vi "UHR-Fleezers Control (host) -Leonardo 04-2018 V2_sym.vi"(0 "Tab Control":T5(tab)=enum."Trap Control (RF)") -> ()   [LabVIEW 2013] (continued)
                    n952 = call "Write to pump.vi"("string"="start", "VISA resource name"=w1530) -> ()  [unwired: 1 out]
                  }
                  frame #3 {
                    n953 = Wait (ms)(milliseconds to wait=u32 500) -> ()  [unwired: 1 out]
                  }
                  frame #4 {
                    n954 = call "Write to pump.vi"("string"="start", "VISA resource name"=w1534) -> ()  [unwired: 1 out]
                  }
                }
              }
            }
          }
          frame Enabled {
            n955 = call "hamilton_controller_shunt2.vi"("Open?"=w1537, "valve"=enum16{"A", "B", "C", "D", "ALL", "E"}."A", "action"=T21."MOVE VALVE") -> ()  [unwired: 8 in, 1 out]
          }
        }
      }
      event "Inject Valve B": Value Change {
        n956 = event-data() -> ()  [unwired: 7 out]
        n957 = disable-structure shown="Enabled" {
          disable-tunnel: "Inject Valve B" -> [w1540 w1560]
          frame Disabled {
            n958 = local read "Pump write delay (ms)"() -> (w1542:dbl)
            n959 = flat-sequence {
              tunnel: w1541 -> [w1555]
              tunnel: w1542 -> [w1551]
              tunnel: w1540 -> [_]
              tunnel: w1542 -> [w1557]
              tunnel: w1541 -> [w1558]
              frame #0 {
                n960 = local read "All Pump Parameters"() -> (w1550:T6)
                n961 = Multiply(x=60.0, y="Flush Center Ch Rate (ul/m)") -> (x*y=w1547:dbl)
                n962 = Unbundle By Name(w1550) -> ("Pump 2"=w1556:T33)
                n963 = call "Set pump parameters.vi"("Pump write delay (ms)"=w1551, "Volume (uL)"="Flush Center Ch Volume (uL)", "Rate (uL/h)"=w1547, "Units"=3.0, "Pump #"=2.0, "Pump Parameters In"=w1556, "VISA resource name"=w1555) -> ("Pump Parameters Out"=w1549:T33)  [unwired: 3 in]
                n964 = Bundle By Name(cluster=w1550, "Pump 2"=w1549) -> (w1548:T6)
                n965 = local write "All Pump Parameters"(w1548) -> ()
                n966 = Add(x="Flush Center Ch Volume (uL)", y="Total Volume\nFlushed (uL)") -> (x+y=w1544:dbl)
                n967 = local write "Total Volume\nFlushed (uL)"(w1544) -> ()
              }
              frame #1 {
                n968 = Wait (ms)(milliseconds to wait=w1557) -> ()  [unwired: 1 out]
              }
              frame #2 {
                n969 = call "Write to pump.vi"("string"="start", "VISA resource name"=w1558) -> ()  [unwired: 1 out]
              }
            }
            n970 = local read "Chemyx Syringe Pump Serial Port"() -> (w1541:refnum<visa-resource-name>)
          }
          frame Enabled {
            n971 = call "hamilton_controller.vi"("Open?"=w1560, "valve"=enum16{"A", "B", "C", "D", "ALL"}."B", "action"=T21."MOVE VALVE") -> ()  [unwired: 8 in, 1 out]
          }
        }
      }
      event "Inject Bottom": Value Change {
        n972 = event-data() -> ()  [unwired: 7 out]
        n973 = call "hamilton_controller_shunt2.vi"("Open?"="Inject Bottom", "valve"=enum16{"A", "B", "C", "D", "ALL", "E"}."C", "action"=T21."MOVE VALVE") -> ()  [unwired: 8 in, 1 out]
      }
      event "Shunt:": Value Change {
        n974 = event-data() -> ()  [unwired: 7 out]
        n975 = call "hamilton_controller_shunt2.vi"("Open?"="Shunt:", "valve"=enum16{"A", "B", "C", "D", "ALL", "E"}."D", "action"=T21."MOVE VALVE") -> ()  [unwired: 8 in, 1 out]
      }
      event "Shunt 2:   2": Value Change {
        n976 = event-data() -> ()  [unwired: 7 out]
        n977 = call "hamilton_controller_shunt2.vi"("Open?"="Shunt 2:   2", "valve"=enum16{"A", "B", "C", "D", "ALL", "E"}."E", "action"=T21."MOVE VALVE") -> ()  [unwired: 8 in, 1 out]
      }
      event "Flip Green Filter": Value Change {
        n978 = event-data() -> ()  [unwired: 7 out]
        n979 = local write "Flip Green Filter"("Flip Green Filter") -> ()
        n980 = flat-sequence {
          tunnel: w1579 -> [w1584]
          tunnel: w1578 -> [w1583]
          tunnel: [w1581] -> w1576
          tunnel: [w1580] -> w1575
          tunnel: [w1586] -> w1574
          tunnel: w1576 -> [w1586]
          tunnel: [w1585] -> w1573
          tunnel: w1575 -> [w1585]
          tunnel: w1574 -> [w1590]
          tunnel: w1573 -> [w1589]
          tunnel: [w1588] -> w1577
          frame #0 {
            n981 = xnode "Read/Write Control"("FPGA VI Reference In"=w1584, "error in"=w1583, "Green Filter Flipper"=TRUE) -> ("FPGA VI Reference Out"=w1581:T20, "error out"=w1580:errorcluster)
          }
          frame #1 {
            n982 = Wait (ms)(milliseconds to wait=u32 100) -> ()  [unwired: 1 out]
          }
          frame #2 {
            n983 = xnode "Read/Write Control"("FPGA VI Reference In"=w1590, "error in"=w1589, "Green Filter Flipper"=FALSE) -> ("error out"=w1588:errorcluster)  [unwired: 1 out]
          }
        }
      }
      event "Pump 1 contents", "Pump 3 contents": Value Change {
        n984 = event-data() -> ()  [unwired: 7 out]
        n985 = local read "Pump 1 contents"() -> (→"Pump 1 cont disp":string)
        n986 = local read "Pump 3 contents"() -> (→"Pump 3 cont disp":string)
      }
      event "Reset Trap Pos. FB": Value Change {
        n987 = event-data() -> ()  [unwired: 7 out]
        n988 = xnode "Read/Write Control"("FPGA VI Reference In"=w1596, "error in"=w1595, "Trap Pos. FB Reset"="Reset Trap Pos. FB") -> ()  [unwired: 2 out]
      }
      event "Trap Pos. FB ON": Value Change {
        n989 = event-data() -> ()  [unwired: 7 out]
        n990 = xnode "Read/Write Control"("FPGA VI Reference In"=w1611, "error in"=w1610) -> ("FPGA VI Reference Out"=w1608:T20, "BD1 Frequency Out 1"=w1605:u64)  [unwired: 1 out]
        n991 = To Double Precision Float(number=w1605) -> (double precision float=w1604:dbl)
        n992 = Multiply(x=49125000.0, y=6.0) -> (x*y=w1603:dbl)
        n993 = Multiply(x=w1604, y=w1603) -> (x*y=w1601:dbl)
        n994 = Scale By Power Of 2(n=-48, x=w1601) -> (x*2^n=w1600:dbl)
        n995 = Divide(x=w1600, y=1000000.0) -> (x/y=w1597:dbl)
        n996 = flat-sequence {
          tunnel: [w1614] -> w1609
          tunnel: w1608 -> [w1615]
          tunnel: w1605 -> [w1613]
          tunnel: "Trap Pos. FB ON" -> [w1612]
          tunnel: "Trap Pos. FB ON" -> [w1621]
          tunnel: w1609 -> [w1620]
          tunnel: "Trap Pos. FB ON" -> [w1623]
          tunnel: w1597 -> [w1622]
          frame #0 {
            n997 = case shown="False" w1612 {
              tunnel: w1615 -> [w1618 w1619]
              tunnel: [w1617 w1619] -> w1614
              tunnel: w1613 -> [w1616 _]
              frame False {
                n998 = xnode "Read/Write Control"("FPGA VI Reference In"=w1618, "BD 1 Frequency 1"=w1616) -> ("FPGA VI Reference Out"=w1617:T20)  [unwired: 1 in, 1 out]
              }
              frame True {
              }
            }
          }
          frame #1 {
            n999 = xnode "Read/Write Control"("FPGA VI Reference In"=w1620, "Force feedback"=w1621) -> ()  [unwired: 1 in, 2 out]
          }
          frame #2 {
            n1000 = case shown="False" w1623 {
              tunnel: w1622 -> [w1626 _]
              frame False {
                n1001 = local read "T2 for asymmetric\n(MHz)"() -> (w1624:dbl)
                n1002 = Subtract(x=w1624, y=w1626) -> (x-y=w1625:dbl)
                n1003 = property on="Trap Delta (MHz)" class="DigNum (strict)"("Val(Sgnl)"=w1625) -> ()  [unwired: 2 in, 2 out]
              }
              frame True {
              }
            }
          }
        }
      }
      event "Diff. FB.", "Trap Pos. FB Gains", "Trap Pos. FB Mult Factor", "Trap Pos. FB Offset Factor", "Trap Pos FB Negate Action", "Trap Pos FB Monitor\nT1 or T2", "Negate Diff?": Value Change {
        n1004 = event-data() -> ()  [unwired: 7 out]
        n1005 = xnode "Read/Write Control"("FPGA VI Reference In"=w1637, "error in"=w1636, "Trap pos. FB Range"="Trap Pos. FB Range", "Trap Pos. FB Gains"="Trap Pos. FB Gains", "Trap Pos. FB Mult Factor"="Trap Pos. FB Mult Factor", "Trap Pos. FB Offset Factor"="Trap Pos. FB Offset Factor", "Trap Pos FB Negate Action"="Trap Pos FB Negate Action", "Trap Pos FB Monitor T1 or T2"="Trap Pos FB Monitor\nT1 or T2", "AI1 X Scale"="Trap Pos. AI1 X Pre-scale", "Negate Diff?"="Negate Diff?", "Diff FB Measurement?"="Diff. FB.") -> ()  [unwired: 2 out]
      }
      event "Trap Pos FB SP": Value Change {
        n1006 = event-data() -> ()  [unwired: 7 out]
        n1007 = xnode "Read/Write Control"("FPGA VI Reference In"=w1640, "error in"=w1639, "Trap Pos. FB SP"="Trap Pos FB SP") -> ()  [unwired: 2 out]
        n1008 = disable-structure shown="Disabled" {
          frame Disabled {
            n1009 = local read "Trap X AI1 (DMA)"() -> (w1661:T13)
            n1010 = local read "Trap X (AI1)"() -> (w1662:T1)
            n1011 = local read "Setpoint offset\nCorrection values"() -> (w1655:dbl[])
            n1012 = local read "Trap Delta (MHz)"() -> (w1659:dbl)
            n1013 = local read "B factor"() -> (w1646:dbl)
            n1014 = Unbundle(w1662) -> ("Trap 1"=w1660:fxp<+/-,16,1>, "Trap 2"=w1649:fxp<+/-,16,1>)
            n1015 = Unbundle(w1661) -> ("Set 1"=w1645:fxp<+/-,16,1>, "Set 2"=w1644:fxp<+/-,16,1>)
            n1016 = Negate(x=w1649) -> (-x=w1642:fxp<+/-,17,2>)
            n1017 = Negate(x=w1660) -> (-x=w1643:fxp<+/-,17,2>)
            n1018 = Divide(x=w1659, y=0.1) -> (x/y=w1657:dbl)
            n1019 = Multiply(x=w1644, y=w1646) -> (x*y=w1647:dbl)
            n1020 = Subtract(x=w1645, y=w1647) -> (x-y=w1652:dbl)
            n1021 = To Long Integer(number=w1657) -> (32bit integer=w1656:i32)
            n1022 = Index Array(array=w1655, index=w1656) -> (element=w1651:dbl)
            n1023 = Multiply(x=w1646, y=w1642) -> (x*y=w1648:dbl)
            n1024 = Subtract(x=w1643, y=w1648) -> (x-y=w1654:dbl)
            n1025 = Add(x=w1654, y=w1651) -> (x+y=→"ideal setpoint fpga":dbl)
            n1026 = Add(x=w1652, y=w1651) -> (x+y=→"ideal setpoint avgd":dbl)
          }
          frame Enabled {
          }
        }
        n1027 = disable-structure shown="Enabled" {
          frame Enabled {
          }
          frame Disabled {
            n1028 = local write "B factor"(1.0 ("B factor")) -> ()
          }
        }
      }
      event "Simulate stepping": Value Change {
        n1029 = event-data() -> ()  [unwired: 7 out]
        n1030 = flat-sequence {
          tunnel: w1664 -> [w1667]
          tunnel: [w1666] -> _
          tunnel: w1663 -> [w1665]
          frame #0 {
            n1031 = while {
              tunnel: w1667 -> [w1695]
              tunnel: [w1694] -> w1666 mode=indexing
              tunnel: w1665 -> [w1693]
              i -> [w1679]
              stop <- w1676 stop-if-true
              w1669 = 1000.0
              n1032 = Divide(x="Backtrack probability", y=100) -> (x/y=w1703:dbl)
              n1033 = Random Number (0-1)() -> (number: 0 to 1=w1704:dbl)
              n1034 = Greater?(x=w1704, y=w1703) -> (0:w1702:bool)
              n1035 = Select(t=1, s=w1702, f=-1) -> (s? t:f=w1699:i32)
              n1036 = local read "BD 1 Frequency 2 (MHz)"() -> (w1674:dbl)
              n1037 = Multiply(x=w1699, y="Step size (nm)") -> (x*y=w1697:dbl)
              "Step taken" <- w1697
              n1038 = Divide(x=w1697, y=168.33) -> (x/y=w1672:dbl)
              n1039 = local read "BD 1 Frequency 1 (MHz)"() -> (w1673:dbl)
              n1040 = local read "X RF Frequency Limits (MHz)"() -> (w1692:T16)
              n1041 = local read "Y RF Frequency Limits (MHz)"() -> (w1691:T16)
              n1042 = Subtract(x=w1673, y=w1672) -> (x-y=w1671:dbl)
              n1043 = local write "BD 1 Frequency 1 (MHz)"(w1671) -> ()
              n1044 = local read "BD 2 Frequency 1 (MHz)"() -> (w1689:dbl)
              n1045 = local read "BD 2 Frequency 2 (MHz)"() -> (w1690:dbl)
              n1046 = call "set RF board frequency - interlace.vi"("Board 2 Frequency Limits"=w1691, "Board 1 Frequency Limits"=w1692, "error in"=w1695, "FPGA VI Reference In"=w1693, "Board 2 Frequency 2 (MHz)"=w1690, "Board 2 Frequency 1 (MHz)"=w1689, "Board 1 Frequency 2 (MHz)"=w1674, "Board 1 Frequency 1  (MHz)"=w1671) -> ("error out"=w1694:errorcluster)  [unwired: 2 in, 1 out]
              n1047 = Subtract(x=w1674, y=w1671) -> (x-y=w1688:dbl)
              n1048 = Subtract(x=w1690, y=w1689) -> (x-y=w1687:dbl)
              n1049 = Square(x=w1687) -> (x^2=w1685:dbl)
              n1050 = Square(x=w1688) -> (x^2=w1686:dbl)
              n1051 = Add(x=w1686, y=w1685) -> (x+y=w1684:dbl)
              n1052 = Square Root(x=w1684) -> (sqrt(x)=w1675:dbl)
              n1053 = local write "Trap Delta (MHz)"(w1675) -> ()
              n1054 = property on="Initial delta (MHz)" class="DigNum (strict)"("Val(Sgnl)"=w1675) -> ()  [unwired: 2 in, 2 out]
              n1055 = Multiply(x="Mean dwell time (s)", y=w1669) -> (x*y=w1681:dbl)
              n1056 = case shown="\"Gamma2\"" "Distribution" {
                tunnel: w1681 -> [w1708 w1712 w1715]
                tunnel: [w1708 w1709 w1716] -> w1670
                frame "uniform", Default {
                }
                frame "Exponential" {
                  n1057 = call-poly <vilib>:"Continuous Random.vi"("b"=w1712, "samples"=1) -> ("exp random data"=w1710:dbl[])  [unwired: 8 in, 1 out]
                  n1058 = Index Array(array=w1710) -> (element=w1709:dbl)  [unwired: 1 in]
                }
                frame "Gamma2" {
                  w1713 = 2.0
                  # "Note: the shape and scale\nparameters of the gamma\nare inverted because LabView..."
                  n1059 = Divide(x=w1715, y=w1713) -> (x/y=w1714:dbl)
                  n1060 = call-poly <vilib>:"Continuous Random.vi"("c"=w1714, "b"=w1713, "samples"=1) -> ("gamma random numbers"=w1717:dbl[])  [unwired: 7 in, 1 out]
                  n1061 = Index Array(array=w1717) -> (element=w1716:dbl)  [unwired: 1 in]
                }
              }
              n1062 = Divide(x=w1670, y=w1669) -> (x/y=→"Step duration":dbl)
              n1063 = To Unsigned Long Integer(number=w1670) -> (unsigned 32bit integer=w1682:u32)
              n1064 = Add(x=w1679, y=1) -> (x+y=w1678:i32)
              n1065 = Wait (ms)(milliseconds to wait=w1682) -> ()  [unwired: 1 out]
              n1066 = Equal?(x=w1678, y="Number of steps") -> (x = y?=w1676:bool)
            }
          }
          frame #1 {
            n1067 = local write "Simulate stepping"(FALSE) -> ()
          }
        }
      }
      event "Set SP to Reading": Value Change {
        n1068 = event-data() -> ()  [unwired: 7 out]
        n1069 = local read "Trap Pos FB Monitor\nT1 or T2"() -> (w1727:bool)
        n1070 = local read "Trap X AI1 (DMA)"() -> (w1730:T13)
        n1071 = local read "Trap X (AI1)"() -> (w1733:T1)
        n1072 = Unbundle By Name(w1733) -> ("Trap 1"=w1732:fxp<+/-,16,1>, "Trap 2"=w1731:fxp<+/-,16,1>)
        n1073 = Unbundle By Name(w1730) -> ("Set 1"=w1729:fxp<+/-,16,1>, "Set 2"=w1728:fxp<+/-,16,1>)
        n1074 = Select(t=w1732, s=w1727, f=w1731) -> (s? t:f=w1726:fxp<+/-,16,1>)
        n1075 = Select(t=w1729, s=w1727, f=w1728) -> (s? t:f=w1725:fxp<+/-,16,1>)
        n1076 = Not(x="Set SP Using...") -> (.not. x?=w1720:bool)
        n1077 = Select(t=w1726, s=w1720, f=w1725) -> (s? t:f=w1721:fxp<+/-,16,1>)
        n1078 = xnode "Read/Write Control"("FPGA VI Reference In"=w1723, "error in"=w1722, "Trap Pos. FB SP"=w1721) -> ()  [unwired: 2 out]
        n1079 = local write "Trap Pos FB SP"(w1721) -> ()
      }
      event "Trap Pos. FB Out Scale 2^n": Value Change {
        n1080 = event-data() -> ()  [unwired: 7 out]
        n1081 = Scale By Power Of 2(n="Trap Pos. FB Out Scale 2^n", x=ext 1.0) -> (x*2^n=w1735:ext)
        n1082 = property on="Trap Pos. FB Mult Factor" class="DigNum (strict)"("Val(Sgnl)"=w1735) -> ()  [unwired: 2 in, 2 out]
      }
      event "Trap Pos FB Int Count": Value Change {
        n1083 = event-data() -> ()  [unwired: 7 out]
        n1084 = xnode "Read/Write Control"("FPGA VI Reference In"=w1740, "error in"=w1739, "Trap Pos FB Int Count"="Trap Pos FB Int Count") -> ()  [unwired: 2 out]
      }
      event "Target Force (pN)", "Setpoint offset\nCorrection values", "Raster target force (pN)": Value Change {
        w1749 = 2.0
        n1085 = event-data() -> ()  [unwired: 7 out]
        n1086 = disable-structure "Removed B Factor to improve position feedback - Alex 081418 1of3" shown="Enabled" {
          disable-tunnel: [w1779 fxp<+/-,32,16> 1.0 ("B factor")] -> w1741
          frame Disabled {
            n1087 = local read "B factor"() -> (w1780:dbl)
            n1088 = To Fixed-Point(number=w1780) -> (fixed-point=w1779:fxp<+/-,16,16>)  [unwired: 1 in]
          }
          frame Enabled {
          }
        }
        n1089 = xnode "Read/Write Control"("FPGA VI Reference In"=w1743, "B factor"=w1741) -> ("BD1 Frequency Out 1"=w1770:u64)  [unwired: 1 in, 2 out]
        n1090 = local read "BD 1 Frequency 2 (MHz)"() -> (w1769:dbl)
        n1091 = local read "Target Force (pN)"() -> (w1755:dbl)
        n1092 = To Double Precision Float(number=w1770) -> (double precision float=w1776:dbl)
        n1093 = Multiply(x=49125000.0, y=6.0) -> (x*y=w1775:dbl)
        n1094 = Multiply(x=w1776, y=w1775) -> (x*y=w1773:dbl)
        n1095 = Scale By Power Of 2(n=-48, x=w1773) -> (x*2^n=w1772:dbl)
        n1096 = Divide(x=w1772, y=1000000.0) -> (x/y=w1768:dbl)
        n1097 = Subtract(x=w1769, y=w1768) -> (x-y=w1767:dbl)
        n1098 = local read "T1 kappa_x (pN/nm)"() -> (w1756:dbl)
        n1099 = local read "T1 alpha_x (nm/V)"() -> (w1757:dbl)
        n1100 = local read "Negate offset difference"() -> (w1758:bool)
        n1101 = local read "Offset file step size"() -> (w1766:dbl)
        n1102 = Multiply(x="Raster target force (pN)", y=w1749) -> (x*y=w1748:dbl)
        n1103 = Multiply(x=w1755, y=w1749) -> (x*y=w1754:dbl)
        n1104 = local read "Setpoint offset\nCorrection values"() -> (w1763:dbl[])
        n1105 = Divide(x=w1767, y=w1766) -> (x/y=w1765:dbl)
        n1106 = Select(t=-1, s=w1758, f=1) -> (s? t:f=w1759:i32)
        n1107 = To Long Integer(number=w1765) -> (32bit integer=w1764:i32)
        n1108 = Multiply(x=w1757, y=w1756) -> (x*y=w1747:dbl)
        n1109 = Divide(x=w1754, y=w1747) -> (x/y=w1753:dbl)
        n1110 = Index Array(array=w1763, index=w1764) -> (element=w1762:dbl)
        n1111 = Divide(x=w1748, y=w1747) -> (x/y=w1746:dbl)
        n1112 = Multiply(x=w1759, y=w1762) -> (x*y=w1745:dbl)
        n1113 = Add(x=w1753, y=w1745) -> (x+y=w1752:dbl)
        n1114 = Add(x=w1746, y=w1745) -> (x+y=w1744:dbl)
        n1115 = To Fixed-Point(number=w1744) -> (fixed-point=w1742:fxp<+/-,16,1>)  [unwired: 1 in]
        n1116 = To Fixed-Point(number=w1752) -> (fixed-point=w1751:fxp<+/-,16,1>)  [unwired: 1 in]
        n1117 = property on="Trap Pos FB SP" class="DigNum (strict)"("Val(Sgnl)"=w1751) -> ()  [unwired: 2 in, 2 out]
        n1118 = xnode "Read/Write Control"("FPGA VI Reference In"=w1743, "Raster setpoint"=w1742) -> ()  [unwired: 1 in, 2 out]
      }
      event "Read setpoint correction\nfile": Value Change {
        n1119 = event-data() -> ()  [unwired: 7 out]
        n1120 = local write "Read setpoint correction\nfile"(FALSE) -> ()
        n1121 = Open/Create/Replace File(file path (use dialog)="Setpoint correction\noffset file", operation (0:open)=T24."open", access (0:read/write)=enum16{"read/write", "read-only", "write-only"}."read-only") -> (refnum out=w1807:refnum<file>)  [unwired: 1 in, 4 out]
        n1122 = Deny Access(7:w1807) -> (3:w1805:refnum<file>)  [unwired: 1 in, 2 out]
        n1123 = Read from Binary File(5:0.0, 9:T30."big-endian, network order" ("byte order (0:big-endian, network order)"), 10:-1 ("count (1)"), 11:w1805) -> (2:w1798:dbl[], 3:w1804:refnum<file>)  [unwired: 1 in, 3 out]
        n1124 = Close File(refnum=w1804) -> ()  [unwired: 1 in, 2 out]
        n1125 = Index Array(array=w1798, index=0) -> (element=w1794:dbl)
        n1126 = local write "Offset file step size"(w1794) -> ()
        n1127 = Array Subset(array=w1798, index=3) -> (w1797:dbl[])  [unwired: 1 in]
        n1128 = local read "T1 kappa_x (pN/nm)"() -> (w1792:dbl)
        n1129 = local read "T1 alpha_x (nm/V)"() -> (w1793:dbl)
        n1130 = local read "T2 alpha_x (nm/V)"() -> (w1791:dbl)
        n1131 = local read "T2 kappa_x (pN/nm)"() -> (w1790:dbl)
        n1132 = Decimate 1D Array(w1797) -> (w1786:dbl[], w1787:dbl[])  [unwired: 1 out]
        n1133 = local read "Offset Values"() -> (w1796:T14)
        n1134 = Multiply(x=w1793, y=w1792) -> (x*y=w1788:dbl)
        n1135 = Multiply(x=w1791, y=w1790) -> (x*y=w1789:dbl)
        n1136 = Bundle By Name(cluster=w1796, "Trap 1X offset"=w1786, "Trap 2X offset"=w1787) -> (w1795:T14)
        n1137 = Divide(x=w1789, y=w1788) -> (x/y=w1783:dbl)
        n1138 = disable-structure "Removed B Factor to better position FB - Alex 081418 3of3" shown="Enabled" {
          disable-tunnel: w1783 -> [w1811 _]
          disable-tunnel: [w1811 1.0] -> w1782
          frame Disabled {
          }
          frame Enabled {
          }
        }
        n1139 = Multiply(x=w1787, y=w1782) -> (x*y=w1785:dbl[])
        n1140 = local write "Offset Values"(w1795) -> ()
        n1141 = Subtract(x=w1786, y=w1785) -> (x-y=w1784:dbl[])
        n1142 = property on="B factor" class="DigNum (strict)"("Val(Sgnl)"=w1782) -> ()  [unwired: 2 in, 2 out]
        n1143 = property on="Setpoint offset\nCorrection values" class="Arr (strict)"("Val(Sgnl)"=w1784) -> ()  [unwired: 2 in, 2 out]
      }
      event "MCL Tracking": Value Change {
        n1144 = event-data() -> ()  [unwired: 7 out]
        n1145 = case shown="True" "MCL Tracking" {
          frame False {
            n1146 = local read "Current MCL (V)"() -> (w1814:dbl)
            n1147 = local write "AO2"(w1814) -> ()
          }
          frame True {
            n1148 = local read "BD 1 Frequency 1 (MHz)"() -> (→"Zero T1 position":dbl)
            n1149 = local read "AO2"() -> (→"Zero MCL x position":dbl)
          }
        }
      }
      event "Scale intensities": Value Change {
        n1150 = event-data() -> ()  [unwired: 7 out]
        n1151 = local read "Trap Intensity\nSetpoints (V)"() -> (w1820:cluster{"Set 1":dbl, "Set 2":dbl})
        n1152 = local read "T1 kappa_x (pN/nm)"() -> (w1826:dbl)
        n1153 = local read "T2 kappa_x (pN/nm)"() -> (w1825:dbl)
        n1154 = Unbundle By Name(w1820) -> ("Set 1"=w1822:dbl, "Set 2"=w1821:dbl)
        n1155 = case shown="True" "Scale intensities" {
          tunnel: "Scale factor" -> [w1836 w1848]
          tunnel: "Scale factor" -> [w1831 w1841]
          tunnel: w1826 -> [w1838 w1847]
          tunnel: w1825 -> [w1837 w1846]
          tunnel: [w1834 w1845] -> w1824
          tunnel: [w1835 w1844] -> w1823
          tunnel: w1822 -> [w1833 w1843]
          tunnel: w1821 -> [w1832 w1842]
          tunnel: [w1830 w1840] -> w1819
          tunnel: [w1829 w1839] -> w1818
          frame False {
            n1156 = Divide(x=w1838, y=w1831) -> (x/y=w1834:dbl)
            n1157 = Divide(x=w1837, y=w1836) -> (x/y=w1835:dbl)
            n1158 = Divide(x=w1833, y=w1831) -> (x/y=w1830:dbl)
            n1159 = Divide(x=w1832, y=w1831) -> (x/y=w1829:dbl)
          }
          frame True {
            n1160 = Multiply(x=w1843, y=w1841) -> (x*y=w1840:dbl)
            n1161 = Multiply(x=w1842, y=w1841) -> (x*y=w1839:dbl)
            n1162 = Multiply(x=w1847, y=w1841) -> (x*y=w1845:dbl)
            n1163 = Multiply(x=w1848, y=w1846) -> (x*y=w1844:dbl)
          }
        }
        n1164 = local write "T2 kappa_x (pN/nm)"(w1823) -> ()
        n1165 = local write "T1 kappa_x (pN/nm)"(w1824) -> ()
        n1166 = Bundle By Name(cluster=w1820, "Set 1"=w1819, "Set 2"=w1818) -> (w1817:cluster{"Set 1":dbl, "Set 2":dbl})
        n1167 = property on="Trap Intensity\nSetpoints (V)" class="Clust (strict)"("Val(Sgnl)"=w1817) -> ()  [unwired: 2 in, 2 out]
      }
    }
    "error out 2" <- w772
    n1168 = node-c288() -> ()  [unwired: 1 in, 1 out]
  }
  n1169 = node-c288() -> (w103:T25)  [unwired: 4 in]
  n1170 = timed-loop "Run Scripts, including: stage motion" {
    timing: w103 -> [_]
    timing-out: [_] -> w102
    tunnel: w61 -> [_]
    stop <- w1850 stop-if-true
    n1171 = node-c288() -> ()  [unwired: 1 in, 1 out]
    n1172 = event shown="[8] \"Take Stepping Data\": Value Change" {
      selector: _ -> [_ _ _ _ _ _ _ _ _ _ _ _]
      dyn-events: _ -> [_ _ _ _ _ _ _ _ _ _ _ _]
      timeout: 50 -> [_ _ _ _ _ _ _ _ _ _ _ _]
      tunnel: ["Move Cap. 1 (DNA Top)" _ "Cal/Data Acq. Spot" "Dump Beads" "Dip for Protein" _ "Got ADig bead" "Got DNA bead" "Take Stepping Data" _ "Take Detection Laser\nImage" _] -> _
      tunnel: [_ _ _ _ _ _ _ _ _ _ _ w2060] -> w1850
      event "Move Cap. 1 (DNA Top)": Value Change {
        n1173 = event-data() -> ()  [unwired: 1 in, 5 out]
        n1174 = local write "Move Cap. 1 (DNA Top)"(FALSE ("Move Cap. 1 (DNA Right)")) -> ()
        n1175 = flat-sequence {
          tunnel: "Cap 1 Samp Flow ON" -> [w1856]
          frame #0 {
            n1176 = local write "Stage Moving"(FALSE ("Stage Moving")) -> ()
            n1177 = case "stop flow" shown="True" w1856 {
              frame False {
              }
              frame True {
                n1178 = call "hamilton_controller.vi"("Open?"=FALSE, "valve"=enum16{"A", "B", "C", "D", "ALL"}."C", "action"=T21."MOVE VALVE") -> ()  [unwired: 8 in, 1 out]
              }
            }
            n1179 = case shown="True" TRUE {
              tunnel: "Cap 1 T ON" -> [w1865 w1866]
              frame False {
                n1180 = property on="Trap 1 (ON/OFF)" class="Bool (strict)"("Val(Sgnl)"=w1865) -> ()  [unwired: 2 in, 2 out]
              }
              frame True {
                n1181 = property on="Trap 2 (ON/OFF)" class="Bool (strict)"("Val(Sgnl)"=w1866) -> ()  [unwired: 2 in, 2 out]
              }
            }
            n1182 = call <vilib>:"Beep.vi"() -> ()  [unwired: 3 in, 9 out]
            n1183 = case shown="True" "Cap 1 Flow ON" {
              frame False {
              }
              frame True {
                n1184 = property on="Main:" class="Bool (strict)"("Val(Sgnl)"=TRUE ("Value (Signaling)")) -> ()  [unwired: 2 in, 2 out]
              }
            }
          }
        }
      }
      event Timeout {
        n1185 = event-data() -> ()  [unwired: 1 in, 2 out]
      }
      event "Cal/Data Acq. Spot": Value Change {
        # "wait for calibration file\nto be written"
        # "signal save cal true\nthis tells the data \nacquisition loop to\nstart sending the data\nto a calibration file"
        # "separate traps to\nthe desired trap delta"
        # "move stage to data acquisition spot"
        # "CHANGE FISH FOR TETHER BACK\nTO TRUE VALUE HERE."
        n1186 = event-data() -> ()  [unwired: 1 in, 5 out]
        n1187 = flat-sequence {
          tunnel: ["Cal @ (MHz)"] -> w1867
          tunnel: w1867 -> [w1879]
          tunnel: w1867 -> [w1900]
          frame #0 {
            n1188 = property on="Trap Delta (MHz)" class="DigNum (strict)"("Val(Sgnl)"="Cal @ (MHz)") -> ()  [unwired: 2 in, 2 out]
            n1189 = call <vilib>:"Beep.vi"() -> ()  [unwired: 3 in, 9 out]
          }
          frame #1 {
            n1190 = local read "Scale intensities"() -> (w1871:bool)
            n1191 = case shown="True" w1871 {
              frame False {
              }
              frame True {
                n1192 = property on="Scale intensities" class="Bool (strict)"("Val(Sgnl)"=FALSE ("Value (Signaling)")) -> ()  [unwired: 2 in, 2 out]
              }
            }
          }
          frame #2 {
            n1193 = Wait (ms)(milliseconds to wait=u32 500) -> ()  [unwired: 1 out]
          }
          frame #3 {
            n1194 = property on="Save Calibration" class="Bool (strict)"("Val(Sgnl)"=TRUE ("Value (Signaling)")) -> ()  [unwired: 2 in, 2 out]
          }
          frame #4 {
            n1195 = Wait (ms)(milliseconds to wait=u32 4000) -> ()  [unwired: 1 out]
          }
          frame #5 {
            n1196 = while {
              stop <- w1876 stop-if-true
              n1197 = local read "Saving..."() -> (w1877:bool)
              n1198 = Wait (ms)(milliseconds to wait=u32 100) -> ()  [unwired: 1 out]
              n1199 = Not(x=w1877) -> (.not. x?=w1876:bool)
            }
          }
          frame #6 {
            n1200 = case shown="True" "W/ Offset 1" {
              tunnel: w1879 -> [_ w1881]
              frame False {
              }
              frame True {
                n1201 = stacked-sequence {
                  tunnel: w1881 -> [_ _ _ _ _ _ _ w1898]
                  frame #0 {
                    n1202 = Replace Array Subset(array=u32[] [0] ("Index Values"), new element="Offset 1 Set", index=0) -> (w1882:u32[])
                    n1203 = property on="Saved AOD Raster Scan Parameter Sets" class="Arr (strict)"("Index Values"=w1882) -> ()  [unwired: 2 in, 2 out]
                    n1204 = property on="Trap Delta (MHz)" class="DigNum (strict)"("Val(Sgnl)"="Offset 1 Start (MHz)") -> ()  [unwired: 2 in, 2 out]
                  }
                  frame #1 {
                    n1205 = Wait (ms)(milliseconds to wait=u32 200) -> ()  [unwired: 1 out]
                  }
                  frame #2 {
                    n1206 = property on="Load parameters" class="Bool (strict)"("Val(Sgnl)"=TRUE ("Value (Signaling)")) -> ()  [unwired: 2 in, 2 out]
                  }
                  frame #3 {
                    n1207 = Wait (ms)(milliseconds to wait=u32 200) -> ()  [unwired: 1 out]
                  }
                  frame #4 {
                    n1208 = property on="Trap Raster Scan" class="Bool (strict)"("Val(Sgnl)"=TRUE ("Value (Signaling)")) -> ()  [unwired: 2 in, 2 out]
                  }
                  frame #5 {
                    n1209 = Wait (ms)(milliseconds to wait=u32 2000) -> ()  [unwired: 1 out]
                  }
                  frame #6 {
                    n1210 = while {
                      stop <- w1895 stop-if-true
                      n1211 = local read "Raster Scanning..."() -> (w1897:bool)
                      n1212 = local read "Saving..."() -> (w1893:bool)
                      n1213 = Wait (ms)(milliseconds to wait=u32 100) -> ()  [unwired: 1 out]
                      n1214 = Not(x=w1893) -> (.not. x?=w1892:bool)
                      n1215 = Not(x=w1897) -> (.not. x?=w1894:bool)
                      n1216 = And(x=w1894, y=w1892) -> (x .and. y?=w1895:bool)
                    }
                  }
                  frame #7 {
                    n1217 = property on="Trap Delta (MHz)" class="DigNum (strict)"("Val(Sgnl)"=w1898) -> ()  [unwired: 2 in, 2 out]
                  }
                }
              }
            }
          }
          frame #7 {
            n1218 = local read "Save ave N"() -> (w1899:dbl)
            n1219 = case shown="True" "W/ Offset 2" {
              tunnel: w1900 -> [_ w1906]
              tunnel: w1899 -> [_ w1905]
              frame False {
                n1220 = Multiply(x="Cal read wait (s)", y=u32 1000 ("milliseconds to wait")) -> (x*y=w1903:u32)
                n1221 = Wait (ms)(milliseconds to wait=w1903) -> ()  [unwired: 1 out]
              }
              frame True {
                n1222 = stacked-sequence {
                  tunnel: w1906 -> [_ _ _ _ _ _ _ _ _ w1927 _ _]
                  tunnel: w1905 -> [_ _ _ _ _ _ _ _ _ w1925 _ _]
                  frame #0 {
                    n1223 = property on="Save ave N" class="DigNum (strict)"("Val(Sgnl)"=1.0 ("Value (Signaling)")) -> ()  [unwired: 2 in, 2 out]
                  }
                  frame #1 {
                    n1224 = Wait (ms)(milliseconds to wait=u32 500) -> ()  [unwired: 1 out]
                  }
                  frame #2 {
                    n1225 = property on="Trap Delta (MHz)" class="DigNum (strict)"("Val(Sgnl)"="Offset 2 Start (MHz)") -> ()  [unwired: 2 in, 2 out]
                    n1226 = Replace Array Subset(array=u32[] [0] ("Index Values"), new element="Offset 2 Set", index=0) -> (w1911:u32[])
                    n1227 = property on="Saved AOD Raster Scan Parameter Sets" class="Arr (strict)"("Index Values"=w1911) -> ()  [unwired: 2 in, 2 out]
                  }
                  frame #3 {
                    n1228 = Wait (ms)(milliseconds to wait=u32 500) -> ()  [unwired: 1 out]
                  }
                  frame #4 {
                    n1229 = property on="Load parameters" class="Bool (strict)"("Val(Sgnl)"=TRUE ("Value (Signaling)")) -> ()  [unwired: 2 in, 2 out]
                  }
                  frame #5 {
                    n1230 = Wait (ms)(milliseconds to wait=u32 500) -> ()  [unwired: 1 out]
                  }
                  frame #6 {
                    n1231 = property on="Trap Raster Scan" class="Bool (strict)"("Val(Sgnl)"=TRUE ("Value (Signaling)")) -> ()  [unwired: 2 in, 2 out]
                  }
                  frame #7 {
                    n1232 = Wait (ms)(milliseconds to wait=u32 2000) -> ()  [unwired: 1 out]
                  }
                  frame #8 {
                    n1233 = while {
                      stop <- w1920 stop-if-true
                      n1234 = local read "Raster Scanning..."() -> (w1923:bool)
                      n1235 = local read "Saving..."() -> (w1921:bool)
                      n1236 = Wait (ms)(milliseconds to wait=u32 100) -> ()  [unwired: 1 out]
                      n1237 = Not(x=w1921) -> (.not. x?=w1919:bool)
                      n1238 = Not(x=w1923) -> (.not. x?=w1922:bool)
                      n1239 = And(x=w1922, y=w1919) -> (x .and. y?=w1920:bool)
                    }
                  }
                  frame #9 {
                    n1240 = property on="Trap Delta (MHz)" class="DigNum (strict)"("Val(Sgnl)"=w1927) -> ()  [unwired: 2 in, 2 out]
                    n1241 = property on="Saved AOD Raster Scan Parameter Sets" class="Arr (strict)"("Index Values"=u32[] [0]) -> ()  [unwired: 2 in, 2 out]
                    n1242 = property on="Save ave N" class="DigNum (strict)"("Val(Sgnl)"=w1925) -> ()  [unwired: 2 in, 2 out]
                  }
                  frame #10 {
                    n1243 = Wait (ms)(milliseconds to wait=u32 500) -> ()  [unwired: 1 out]
                  }
                  frame #11 {
                    n1244 = property on="Load parameters" class="Bool (strict)"("Val(Sgnl)"=TRUE ("Value (Signaling)")) -> ()  [unwired: 2 in, 2 out]
                  }
                }
              }
            }
          }
          frame #8 {
            n1245 = property on="Read Cal" class="Bool (strict)"("Val(Sgnl)"=TRUE ("Value (Signaling)")) -> ()  [unwired: 2 in, 2 out]
          }
          frame #9 {
            n1246 = Wait (ms)(milliseconds to wait=u32 500) -> ()  [unwired: 1 out]
          }
          frame #10 {
            n1247 = property on="Fish for Tether" class="Bool (strict)"("Val(Sgnl)"=FALSE ("Value (Signaling)")) -> ()  [unwired: 2 in, 2 out]
          }
        }
        n1248 = local write "Cal/Data Acq. Spot"(FALSE ("Cal/Data Acq. Spot")) -> ()
      }
      event "Dump Beads": Value Change {
        # "SCRIPT TO REMOVE BOTH BEADS FROM THE TRAPS. TURNS ON LIGHT WHICH INDICATES THAT STAGE IS MOVING. THEN STOPS SAVING DATA. \nSETS Sample Channel Flow TO TRUE. STOPS INTERLACING GREEN FLUORESCENCE. TURNS OFF Tether INDICATOR BECAUSE WE ARE THROWING IT\nAWAY. SHUTS OFF TRAP POSITION FEEDBACK."
        n1249 = event-data() -> ()  [unwired: 1 in, 5 out]
        n1250 = flat-sequence {
          frame #0 {
            w1934 = FALSE ("Fl. Triggered...")
            w1935 = TRUE ("Stage Moving")
            n1251 = local read "Saving..."() -> (w1936:bool)
            n1252 = local write "Fl. Triggered..."(w1934) -> ()
            n1253 = local write "Stage Moving"(w1935) -> ()
            n1254 = local write "Tether"(w1934) -> ()
            n1255 = property on="Green Laser ON/Interlacing" class="Bool (strict)"("Val(Sgnl)"=w1934) -> ()  [unwired: 2 in, 2 out]
            n1256 = property on="Trap Pos. FB ON" class="Bool (strict)"("Val(Sgnl)"=w1934) -> ()  [unwired: 2 in, 2 out]
            n1257 = property on="Inject Bottom" class="Bool (strict)"("Val(Sgnl)"=w1935) -> ()  [unwired: 2 in, 2 out]
            n1258 = local write "Stop Saving"(w1936) -> ()
          }
          frame #1 {
            w1937 = FALSE ("Value (Signaling)")
            # "TURNS TRAPS OFF SO THAT\nBEADS REMAIN AT DUMP \nBEADS POSITION"
            n1259 = property on="Trap 1 (ON/OFF)" class="Bool (strict)"("Val(Sgnl)"=w1937) -> ()  [unwired: 2 in, 2 out]
            n1260 = property on="Trap 2 (ON/OFF)" class="Bool (strict)"("Val(Sgnl)"=w1937) -> ()  [unwired: 2 in, 2 out]
            n1261 = call <vilib>:"Beep.vi"() -> ()  [unwired: 3 in, 9 out]
          }
          frame #2 {
            n1262 = property on="Goto Bottom (F7)" class="Bool"("Val(Sgnl)"=TRUE ("Value (Signaling)")) -> ()  [unwired: 2 in, 2 out]
          }
          frame #3 {
            n1263 = Wait (ms)(milliseconds to wait=u32 8000) -> ()  [unwired: 1 out]
          }
          frame #4 {
            n1264 = property on="Trap Delta (MHz)" class="DigNum (strict)"("Val(Sgnl)"=20.0 ("Value (Signaling)")) -> ()  [unwired: 2 in, 2 out]
          }
          frame #5 {
            n1265 = property on="Trap 2 (ON/OFF)" class="Bool (strict)"("Val(Sgnl)"=TRUE ("Value (Signaling)")) -> ()  [unwired: 2 in, 2 out]
          }
          frame #6 {
            n1266 = property on="Inject Bottom" class="Bool (strict)"("Val(Sgnl)"=FALSE ("Value (Signaling)")) -> ()  [unwired: 2 in, 2 out]
          }
        }
      }
      event "Dip for Protein": Value Change {
        n1267 = event-data() -> ()  [unwired: 1 in, 5 out]
        n1268 = flat-sequence {
          frame #0 {
            n1269 = case shown="True" "Move Trap Before?" {
              frame False {
              }
              frame True {
                n1270 = property on="Trap Delta (MHz)" class="DigNum (strict)"("Val(Sgnl)"="Dip Trap Delta 1 (MHz)") -> ()  [unwired: 2 in, 2 out]
              }
            }
          }
          frame #1 {
            n1271 = Multiply(x="Duration (s)", y=1000.0) -> (x*y=w1946:dbl)
            n1272 = Wait (ms)(milliseconds to wait=w1946) -> ()  [unwired: 1 out]
          }
          frame #2 {
            n1273 = case shown="True" "Move Trap After?" {
              frame False {
              }
              frame True {
                n1274 = property on="Trap Delta (MHz)" class="DigNum (strict)"("Val(Sgnl)"="Dip Trap Delta 2 (MHz)") -> ()  [unwired: 2 in, 2 out]
              }
            }
          }
          frame #3 {
            n1275 = case shown="True" "Green ON After?" {
              frame False {
              }
              frame True {
                n1276 = property on="Green Laser ON/Interlacing" class="Bool (strict)"("Val(Sgnl)"=TRUE ("Value (Signaling)")) -> ()  [unwired: 2 in, 2 out]
              }
            }
          }
          frame #4 {
            n1277 = Wait (ms)(milliseconds to wait=u32 500) -> ()  [unwired: 1 out]
          }
          frame #5 {
            n1278 = case shown="True" "Save Data After?" {
              frame False {
              }
              frame True {
                n1279 = property on="Start Saving" class="Bool (strict)"("Val(Sgnl)"=TRUE ("Value (Signaling)")) -> ()  [unwired: 2 in, 2 out]
              }
            }
          }
        }
      }
      event "Profile": Value Change {
        n1280 = event-data() -> ()  [unwired: 1 in, 5 out]
        n1281 = flat-sequence {
          frame #0 {
            w1956 = 0.0 ("element")
            n1282 = Build Array(w1956, "Y change (mm)", w1956) -> ()  [unwired: 1 out]
          }
          frame #1 {
            # "stop saving"
            n1283 = local write "Stop Saving"(TRUE ("Stop Saving")) -> ()
            n1284 = local write "Stage Moving"(FALSE ("Stage Moving")) -> ()
          }
        }
      }
      event "Got ADig bead": Value Change {
        n1285 = event-data() -> ()  [unwired: 1 in, 5 out]
        n1286 = property on="Move Cap. 1 (DNA Top)" class="Bool (strict)"("Val(Sgnl)"=TRUE ("Value (Signaling)")) -> ()  [unwired: 2 in, 2 out]
        n1287 = property on="Inject Top:" class="Bool (strict)"("Val(Sgnl)"=FALSE ("Value (Signaling)")) -> ()  [unwired: 2 in, 2 out]
      }
      event "Got DNA bead": Value Change {
        n1288 = event-data() -> ()  [unwired: 1 in, 5 out]
        n1289 = property on="Cal/Data Acq. Spot" class="Bool (strict)"("Val(Sgnl)"=TRUE ("Value (Signaling)")) -> ()  [unwired: 2 in, 2 out]
        n1290 = property on="Main:" class="Bool (strict)"("Val(Sgnl)"=FALSE ("Value (Signaling)")) -> ()  [unwired: 2 in, 2 out]
      }
      event "Take Stepping Data": Value Change {
        n1291 = event-data() -> ()  [unwired: 1 in, 5 out]
        n1292 = local read "Save ave N"() -> (w1974:dbl)
        n1293 = flat-sequence {
          tunnel: w1974 -> [w1976]
          tunnel: [w1976] -> w1969
          tunnel: [w1978] -> w1970
          tunnel: w1969 -> [w1978]
          tunnel: [w1980] -> w1971
          tunnel: w1970 -> [w1980]
          tunnel: [w1983] -> w1972
          tunnel: w1971 -> [w1983]
          tunnel: [w1985] -> w1973
          tunnel: w1972 -> [w1985]
          tunnel: [w1987] -> w1967
          tunnel: w1973 -> [w1987]
          tunnel: w1967 -> [w1990]
          tunnel: [w1990] -> w1966
          tunnel: w1966 -> [w1991]
          tunnel: [w1991] -> w1968
          tunnel: w1968 -> [w1997]
          frame #0 {
            n1294 = property on="Save ave N" class="DigNum (strict)"("Val(Sgnl)"="Save ave factor") -> ()  [unwired: 2 in, 2 out]
          }
          frame #1 {
            n1295 = Wait (ms)(milliseconds to wait=u32 100) -> ()  [unwired: 1 out]
          }
          frame #2 {
            n1296 = local read "Offset 2 Start (MHz)"() -> (w1982:dbl)
            n1297 = property on="Saved AOD Raster Scan Parameter Sets" class="Arr (strict)"("Index Values"=u32[] [2]) -> ()  [unwired: 2 in, 2 out]
            n1298 = property on="Trap Delta (MHz)" class="DigNum (strict)"("Val(Sgnl)"=w1982) -> ()  [unwired: 2 in, 2 out]
          }
          frame #3 {
            n1299 = property on="Load parameters" class="Bool (strict)"("Val(Sgnl)"=TRUE ("Value (Signaling)")) -> ()  [unwired: 2 in, 2 out]
          }
          frame #4 {
            n1300 = Wait (ms)(milliseconds to wait=u32 100) -> ()  [unwired: 1 out]
          }
          frame #5 {
            n1301 = property on="Trap Raster Scan" class="Bool (strict)"("Val(Sgnl)"=TRUE ("Value (Signaling)")) -> ()  [unwired: 2 in, 2 out]
          }
          frame #6 {
            n1302 = Wait (ms)(milliseconds to wait=u32 1000) -> ()  [unwired: 1 out]
          }
          frame #7 {
            n1303 = while {
              stop <- w1994 stop-if-true
              n1304 = local read "Raster Scanning..."() -> (w1996:bool)
              n1305 = local read "Saving..."() -> (w1995:bool)
              n1306 = Not(x=w1995) -> (.not. x?=w1992:bool)
              n1307 = Not(x=w1996) -> (.not. x?=w1993:bool)
              n1308 = And(x=w1993, y=w1992) -> (x .and. y?=w1994:bool)
            }
          }
          frame #8 {
            n1309 = property on="Save ave N" class="DigNum (strict)"("Val(Sgnl)"=w1997) -> ()  [unwired: 2 in, 2 out]
          }
        }
      }
      event "Step Size (nm)": Value Change {
        n1310 = event-data() -> ()  [unwired: 1 in, 5 out]
        n1311 = flat-sequence {
          frame #0 {
            n1312 = property on="Saved AOD Raster Scan Parameter Sets" class="Arr (strict)"("Index Values"=u32[] [1]) -> ()  [unwired: 2 in, 2 out]
          }
          frame #1 {
            n1313 = Multiply(x="N Steps", y="Step Size (nm)") -> (x*y=w1999:dbl)
            n1314 = property on="Scan Speed AOD (nm/s) 2" class="DigNum (strict)"("Value"="Step Size (nm)") -> ()  [unwired: 2 in, 2 out]
            n1315 = property on="Step Size AOD (nm) 2" class="DigNum (strict)"("Value"="Step Size (nm)") -> ()  [unwired: 2 in, 2 out]
            n1316 = property on="Scan Range AOD (nm) 2" class="DigNum (strict)"("Value"=w1999) -> ()  [unwired: 2 in, 2 out]
          }
        }
      }
      event "Take Detection Laser\nImage": Value Change {
        n1317 = event-data() -> ()  [unwired: 1 in, 5 out]
        n1318 = flat-sequence {
          tunnel: [w2027] -> w2017
          tunnel: [w2026] -> w2010
          tunnel: [w2025] -> w2002
          tunnel: [w2030] -> w2018
          tunnel: w2017 -> [w2030]
          tunnel: [w2029] -> w2011
          tunnel: w2010 -> [w2029]
          tunnel: [w2028] -> w2003
          tunnel: w2002 -> [w2028]
          tunnel: [w2034] -> w2019
          tunnel: w2018 -> [w2034]
          tunnel: [w2033] -> w2012
          tunnel: w2011 -> [w2033]
          tunnel: [w2032] -> w2004
          tunnel: w2003 -> [w2032]
          tunnel: [w2040] -> w2020
          tunnel: w2019 -> [w2040]
          tunnel: [w2039] -> w2013
          tunnel: w2012 -> [w2039]
          tunnel: [w2038] -> w2005
          tunnel: w2004 -> [w2038]
          tunnel: [w2044] -> w2021
          tunnel: w2020 -> [w2044]
          tunnel: [w2043] -> w2014
          tunnel: w2013 -> [w2043]
          tunnel: [w2042] -> w2006
          tunnel: w2005 -> [w2042]
          tunnel: [w2048] -> w2022
          tunnel: w2021 -> [w2048]
          tunnel: [w2047] -> w2015
          tunnel: w2014 -> [w2047]
          tunnel: [w2046] -> w2007
          tunnel: w2006 -> [w2046]
          tunnel: [w2052] -> w2023
          tunnel: w2022 -> [w2052]
          tunnel: [w2051] -> w2016
          tunnel: w2015 -> [w2051]
          tunnel: [w2050] -> w2008
          tunnel: w2007 -> [w2050]
          tunnel: w2023 -> [w2058]
          tunnel: w2016 -> [w2057]
          tunnel: [w2055] -> w2009
          tunnel: w2008 -> [w2055]
          tunnel: w2009 -> [w2059]
          frame #0 {
            n1319 = local read "Green Laser ON/Interlacing"() -> (w2027:bool)
            n1320 = local read "Green laser mode"() -> (w2026:enum32{"Laser ON", "Laser OFF", "Interlace"})
            n1321 = local read "Green FB On/Off"() -> (w2025:bool)
          }
          frame #1 {
            n1322 = property on="Green FB On/Off" class="Bool (strict)"("Val(Sgnl)"=FALSE ("Value (Signaling)")) -> ()  [unwired: 2 in, 2 out]
          }
          frame #2 {
            n1323 = property on="Green Laser ON/Interlacing" class="Bool (strict)"("Val(Sgnl)"=TRUE ("Value (Signaling)")) -> ()  [unwired: 2 in, 2 out]
            n1324 = property on="Flip Green Filter" class="Bool (strict)"("Val(Sgnl)"=TRUE ("Value (Signaling)")) -> ()  [unwired: 2 in, 2 out]
            n1325 = property on="Green laser mode" class="RadioBtnsControl (strict)"("Val(Sgnl)"=enum32{"Laser ON", "Laser OFF", "Interlace"}."Laser ON" ("Value (Signaling)")) -> ()  [unwired: 2 in, 2 out]
          }
          frame #3 {
            n1326 = Wait (ms)(milliseconds to wait=u32 500) -> ()  [unwired: 1 out]
          }
          frame #4 {
            n1327 = property on="Confocal Image" class="Bool (strict)"("Val(Sgnl)"=TRUE ("Value (Signaling)")) -> ()  [unwired: 2 in, 2 out]
          }
          frame #5 {
            n1328 = Wait (ms)(milliseconds to wait=u32 2000) -> ()  [unwired: 1 out]
          }
          frame #6 {
            n1329 = while {
              stop <- w2053 stop-if-true
              n1330 = local read "Saving..."() -> (w2054:bool)
              n1331 = Not(x=w2054) -> (.not. x?=w2053:bool)
            }
          }
          frame #7 {
            n1332 = property on="Flip Green Filter" class="Bool (strict)"("Val(Sgnl)"=TRUE ("Value (Signaling)")) -> ()  [unwired: 2 in, 2 out]
            n1333 = property on="Green Laser ON/Interlacing" class="Bool (strict)"("Val(Sgnl)"=w2058) -> ()  [unwired: 2 in, 2 out]
            n1334 = property on="Green laser mode" class="RadioBtnsControl (strict)"("Val(Sgnl)"=w2057) -> ()  [unwired: 2 in, 2 out]
          }
          frame #8 {
            n1335 = property on="Green FB On/Off" class="Bool (strict)"("Val(Sgnl)"=w2059) -> ()  [unwired: 2 in, 2 out]
          }
        }
      }
      event "Stop All": Value Change {
        n1336 = event-data() -> ()  [unwired: 1 in, 5 out]
        n1337 = local read "Stop All"() -> (w2060:bool)
      }
    }
    n1338 = node-c288() -> ()  [unwired: 1 in, 1 out]
  }
  n1339 = node-c288() -> (w110:T25)  [unwired: 4 out]
  n1340 = timed-loop "Mouse control: trap position (AOM deflection), set confocal spot from image" {
    tunnel: [w2062] -> w70
    tunnel: w61 -> [w2061]
    timing: w110 -> [_]
    timing-out: [_] -> w109
    stop <- w2062 stop-if-true
    n1341 = node-c288() -> ()  [unwired: 2 out]
    n1342 = event shown="[0] \"Pane\": Mouse Down" {
      selector: _ -> [_ _]
      dyn-events: _ -> [_ _]
      timeout: _ -> [_ _]
      tunnel: w2061 -> [w2065 _]
      event Mouse Down {
        n1343 = event-data() -> ("Time"=w2067:u32, "Coords"=w2066:T8, "Button"=w2068:u16)  [unwired: 6 out]
        n1344 = case shown="3" w2068 {
          tunnel: w2067 -> [_ _ w2171]
          tunnel: w2066 -> [_ w2105 w2169]
          tunnel: w2065 -> [_ _ w2167]
          frame 0, Default {
          }
          frame 1 {
            n1345 = property on="APD 2" class="ImageControl"() -> ("Displayed Image Position"=w2075:cluster{"Left":i32, "Top":i32})  [unwired: 2 in, 2 out]
            n1346 = property on="APD 1" class="ImageControl"() -> ("Displayed Image Position"=w2104:cluster{"Left":i32, "Top":i32})  [unwired: 2 in, 2 out]
            n1347 = property on="Detection Laser X" class="ImageControl"() -> ("Displayed Image Position"=w2101:cluster{"Left":i32, "Top":i32})  [unwired: 2 in, 2 out]
            n1348 = property on="Detection Laser Y" class="ImageControl"() -> ("Displayed Image Position"=w2100:cluster{"Left":i32, "Top":i32})  [unwired: 2 in, 2 out]
            n1349 = property on="APD 2" class="ImageControl"() -> ("Displayed Image Size"=w2074:cluster{"Width":u32, "Height":u32})  [unwired: 2 in, 2 out]
            n1350 = property on="APD 1" class="ImageControl"() -> ("Displayed Image Size"=w2102:cluster{"Width":u32, "Height":u32})  [unwired: 2 in, 2 out]
            n1351 = property on="Detection Laser X" class="ImageControl"() -> ("Displayed Image Size"=w2103:cluster{"Width":u32, "Height":u32})  [unwired: 2 in, 2 out]
            n1352 = property on="Detection Laser Y" class="ImageControl"() -> ("Displayed Image Size"=w2099:cluster{"Width":u32, "Height":u32})  [unwired: 2 in, 2 out]
            n1353 = Unbundle By Name(w2074) -> ("Width"=w2071:u32, "Height"=w2070:u32)
            n1354 = Unbundle By Name(w2075) -> ("Left"=w2073:i32, "Top"=w2072:i32)
            n1355 = Unbundle By Name(w2102) -> ("Width"=w2096:u32, "Height"=w2095:u32)
            n1356 = Unbundle By Name(w2103) -> ("Width"=w2092:u32, "Height"=w2091:u32)
            n1357 = Unbundle By Name(w2099) -> ("Width"=w2088:u32, "Height"=w2087:u32)
            n1358 = Unbundle By Name(w2104) -> ("Left"=w2098:i32, "Top"=w2097:i32)
            n1359 = Unbundle By Name(w2101) -> ("Left"=w2094:i32, "Top"=w2093:i32)
            n1360 = Unbundle By Name(w2100) -> ("Left"=w2090:i32, "Top"=w2089:i32)
            n1361 = Bundle("Left"=w2073, "Top"=w2072, "Width"=w2071, "Height"=w2070) -> (w2069:T34)  [unwired: 1 in]
            n1362 = Bundle("Left"=w2098, "Top"=w2097, "Width"=w2096, "Height"=w2095) -> (w2086:T34)  [unwired: 1 in]
            n1363 = Bundle("Left"=w2094, "Top"=w2093, "Width"=w2092, "Height"=w2091) -> (w2085:T34)  [unwired: 1 in]
            n1364 = Bundle("Left"=w2090, "Top"=w2089, "Width"=w2088, "Height"=w2087) -> (w2084:T34)  [unwired: 1 in]
            n1365 = Build Cluster Array(w2069, w2086, w2085, w2084) -> (w2083:T35)
            n1366 = for {
              tunnel: w2105 -> [w2116]
              tunnel: w2083 -> [w2117] mode=indexing
              shift-right: [w2114] -> w2081
              shift-left: TRUE -> [w2115]
              shift-right: [w2113] -> w2079
              shift-left: _ -> [w2109]
              shift-right: [w2112] -> w2078
              shift-left: _ -> [w2108]
              shift-right: [w2111] -> w2077
              shift-left: _ -> [w2107]
              shift-right: [w2110] -> w2076
              shift-left: _ -> [w2106]
              n1367 = case shown="True" w2115 {
                selector: w2115 -> [w2122 _]
                tunnel: w2117 -> [_ w2131]
                tunnel: w2116 -> [_ w2129]
                tunnel: [w2122 w2127] -> w2114
                tunnel: [w2121 w2126] -> w2113
                tunnel: [w2120 w2125] -> w2112
                tunnel: [w2119 w2124] -> w2111
